vi "Polymorphique Simple channel example.vi"() -> ()   [LabVIEW 2020]
uses:
  <userlib>/DAQNavi Polymorphic VI/create/DAQNavi Create Channel(AO-Voltage).vi
  <userlib>/DAQNavi Polymorphic VI/create/DAQNavi Create Channel(AI-Voltage).vi
  <userlib>/DAQNavi Polymorphic VI/write/DAQNavi Write (Analog DBL 1Chan 1Samp).vi
  <userlib>/DAQNavi Polymorphic VI/read/DAQNavi Read (Analog Wfm 1Chan 1Samp).vi
panel:
  in  "Output":dbl=3.0 format="%#_13g"
  out "value range Input":string="+/- 10 V" caption="property value"
  out "physical channels Input":string="DemoDevice,BID#0/ai0:0" caption="property value"
  in  "stop":bool
  out "Waveform Chart":waveform(dbl)(graph)
  out "value range Output":string="+/- 5 V" caption="property value"
  out "physical channels Output":string="DemoDevice, BID#0/ao1:1" caption="property value"
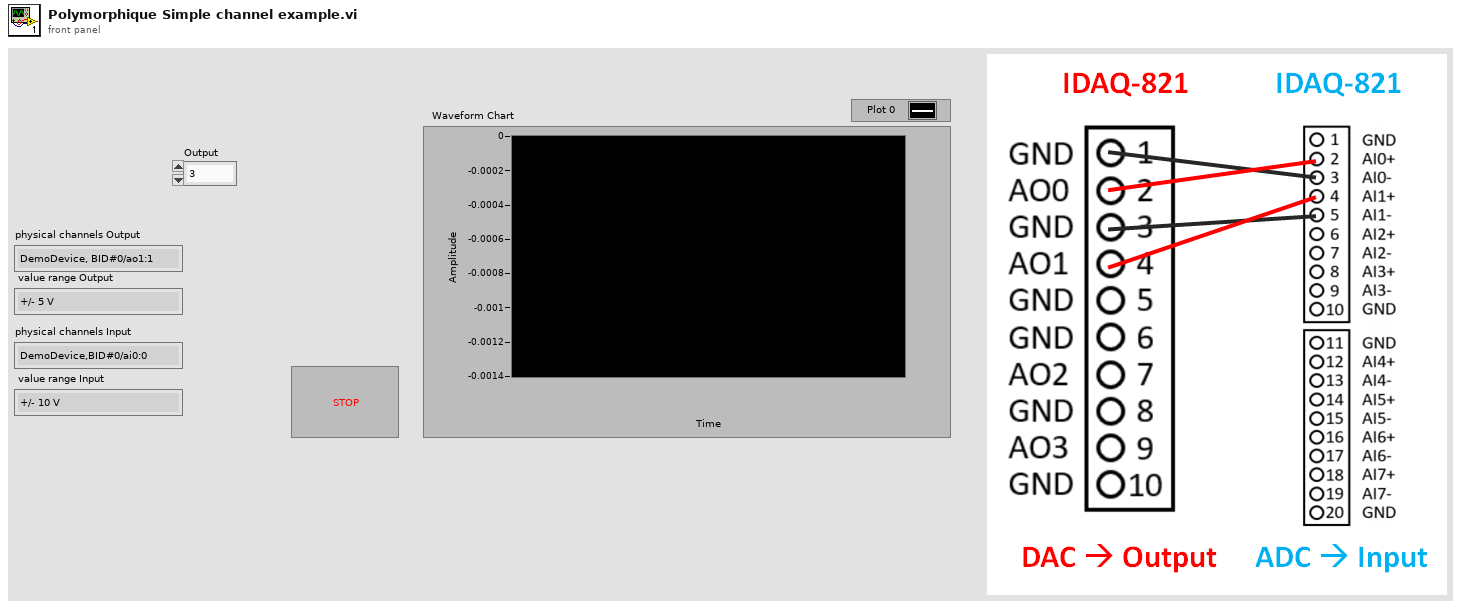
[diagram p1: front panel]
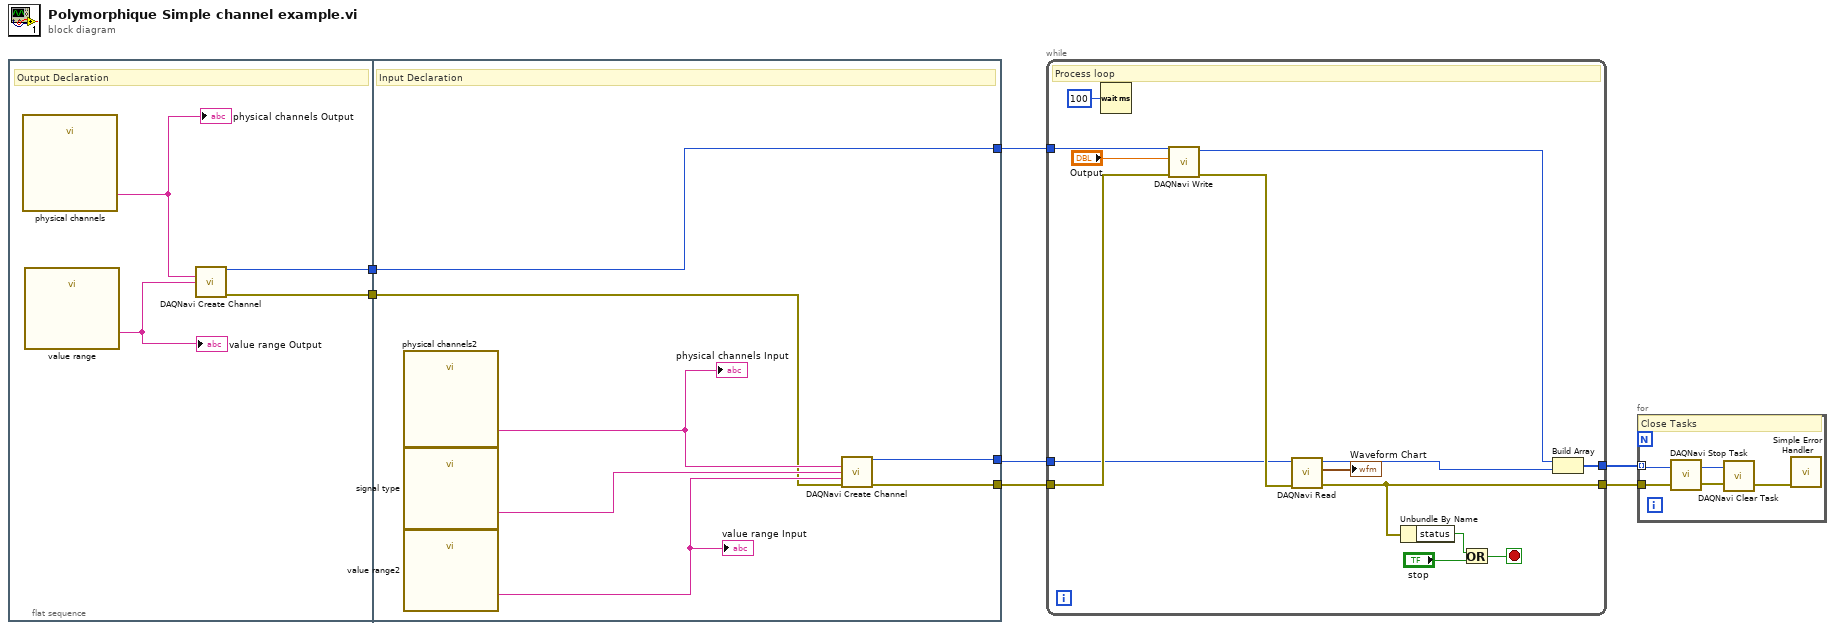
[diagram p0: block diagram]
diagram:
  n1 = flat-sequence {
    tunnel: [w9] -> w7
    tunnel: [w8] -> w6
    tunnel: [w18] -> w5
    tunnel: w7 -> [w14]
    tunnel: w6 -> [w18]
    tunnel: [w13] -> w3
    tunnel: [w12] -> w4
    frame #0 {
      # "Output Declaration"
      n2 = call "physical channels"() -> ("property value"=w10:string)  [unwired: 1 out]
      "physical channels Output" <- w10
      n3 = call "value range"() -> ("property value"=w11:string)  [unwired: 1 out]
      "value range Output" <- w11
      n4 = call-poly <userlib>:"DAQNavi Create Channel.vi"("physical channels"=w10, "value range"=w11) -> ("task out"=w8:i32, "error out"=w9:errorcluster)  [unwired: 3 in, 9 out]
    }
    frame #1 {
      # "Input Declaration"
      n5 = call "physical channels2"() -> ("property value"=w15:string)  [unwired: 1 out]
      "physical channels Input" <- w15
      n6 = call "signal type"() -> ("property value"=w17:string)  [unwired: 1 out]
      n7 = call "value range2"() -> ("property value"=w16:string)  [unwired: 1 out]
      "value range Input" <- w16
      n8 = call-poly <userlib>:"DAQNavi Create Channel.vi"("physical channels"=w15, "signal type"=w17, "value range"=w16, "error in (no error)"=w14) -> ("task out"=w13:i32, "error out"=w12:errorcluster)  [unwired: 1 in, 9 out]
    }
  }
  n9 = while {
    tunnel: w5 -> [w19]
    tunnel: w4 -> [w25]
    tunnel: [w29] -> w1
    tunnel: w3 -> [w20]
    tunnel: [w21] -> w2
    stop <- w31 stop-if-true
    # "Process loop"
    n10 = Wait (ms)(milliseconds to wait=u32 100) -> ()  [unwired: 1 out]
    n11 = call-poly <userlib>:"DAQNavi Write.vi"("error in (no error)"=w25, "data"="Output", "task in"=w19) -> ("error out"=w24:errorcluster, "task out"=w22:i32)  [unwired: 1 in, 6 out]
    n12 = call-poly <userlib>:"DAQNavi Read.vi"("error in (no error)"=w24, "task in"=w20) -> ("error out"=w29:errorcluster, "data"=→"Waveform Chart":waveform(dbl), "task out"=w23:i32)  [unwired: 2 in, 5 out]
    n13 = Unbundle By Name(w29) -> ("status"=w28:bool)
    n14 = Or(x=w28, y="stop") -> (x .or. y?=w31:bool)
    n15 = Build Array(w22, w23) -> (w21:i32[])
  }
  n16 = for {
    tunnel: w2 -> [w35] mode=indexing
    tunnel: w1 -> [w36]
    # "Close Tasks"
    n17 = call <userlib>:"DAQNavi Stop Task.vi"("error in (no error)"=w36, "task in"=w35) -> ("error out"=w33:errorcluster, "task out"=w34:i32)
    n18 = call <userlib>:"DAQNavi Clear Task.vi"("error in (no error)"=w33, "task in"=w34) -> ("error out"=w37:errorcluster)  [unwired: 1 out]
    n19 = call <vilib>:"Simple Error Handler.vi"("error in (no error)"=w37) -> ()  [unwired: 2 in, 7 out]
  }
